vi "TracePartialSnap.vi"() -> ()   [LabVIEW 2012]
uses:
  <vilib>/userdefined/High Color/IMAQdx.ctl
  <vilib>/vision/driver/NI_Vision_Acquisition_Software.lvlib
  <vilib>/vision/NI_Vision_Development_Module.lvlib
panel:
  out "Array":i32[](array[numeric])
  out "Image Out":T1(plugin-control)
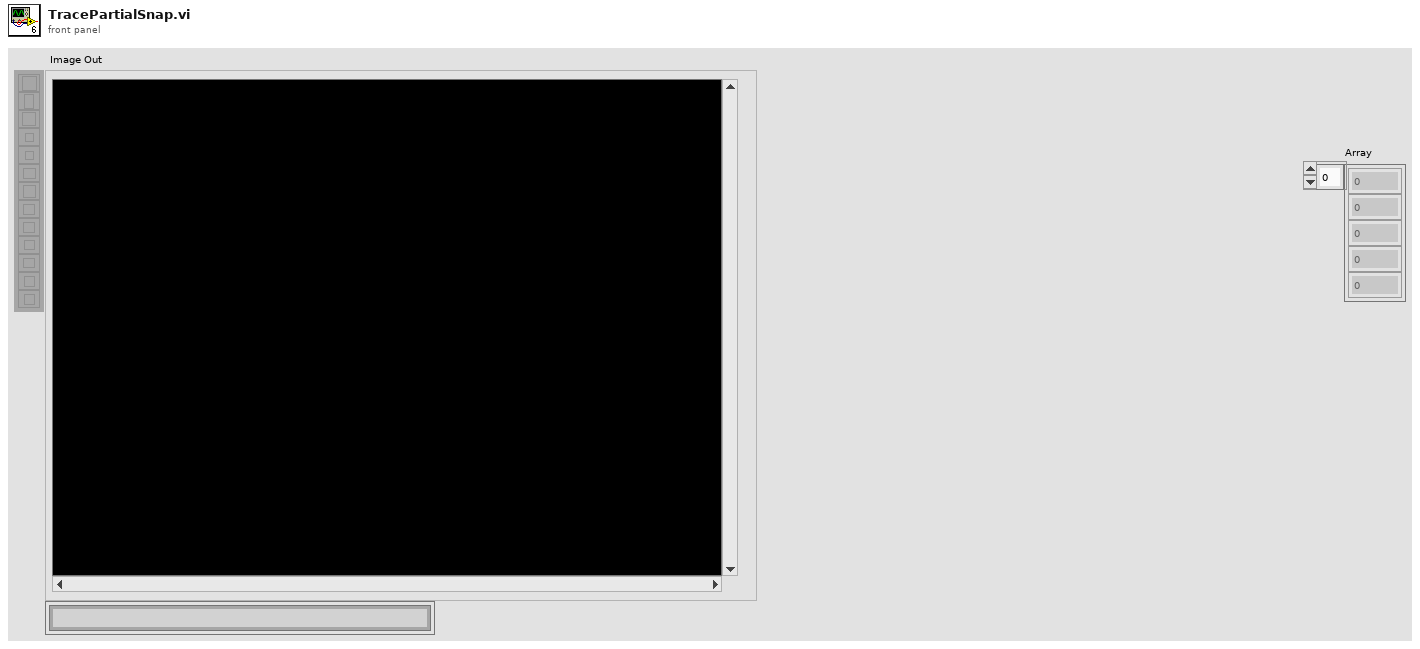
[diagram p1: front panel]
types:
  T1 = typedef "IMAQ Image.ctl" = refnum<image>
  T2 = typedef "Image Type" = u32
  T3 = typedef "IMAQdx.ctl" = refnum<k21>
  T4 = cluster{"Position":cluster{"x":sgl, "y":sgl}, "Angle":sgl, "Scale":sgl, "Score":sgl, "Bounding Box":cluster{"x":sgl, "y":sgl}[]}[]
  T5 = cluster{"Matches (Pattern Matching 1)[0]":cluster{"Position":cluster{"x":sgl, "y":sgl}, "Angle":sgl, "Scale":sgl, "Score":sgl, "Bounding Box":cluster{"x":sgl, "y":sgl}[]}, "Matches (Pattern Matching 1)[1]":cluster{"Position":cluster{"x":sgl, "y":sgl}, "Angle":sgl, "Scale":sgl, "Score":sgl, "Bounding Box":cluster{"x":sgl, "y":sgl}[]}, "Matches (Pattern Matching 1)[2]":cluster{"Position":cluster{"x":sgl, "y":sgl}, "Angle":sgl, "Scale":sgl, "Score":sgl, "Bounding Box":cluster{"x":sgl, "y":sgl}[]}, "Matches (Pattern Matching 1)[3]":cluster{"Position":cluster{"x":sgl, "y":sgl}, "Angle":sgl, "Scale":sgl, "Score":sgl, "Bounding Box":cluster{"x":sgl, "y":sgl}[]}}
  T6 = cluster{"Bounding Box[0]":cluster{"x":sgl, "y":sgl}, "Bounding Box[1]":cluster{"x":sgl, "y":sgl}, "Bounding Box[2]":cluster{"x":sgl, "y":sgl}, "Bounding Box[3]":cluster{"x":sgl, "y":sgl}, "Bounding Box[4]":cluster{"x":sgl, "y":sgl}, "Bounding Box[5]":cluster{"x":sgl, "y":sgl}, "Bounding Box[6]":cluster{"x":sgl, "y":sgl}, "Bounding Box[7]":cluster{"x":sgl, "y":sgl}, "Bounding Box[8]":cluster{"x":sgl, "y":sgl}}
  T7 = cluster{"[0]":i32, "[1]":i32, "[2]":i32, "[3]":i32}
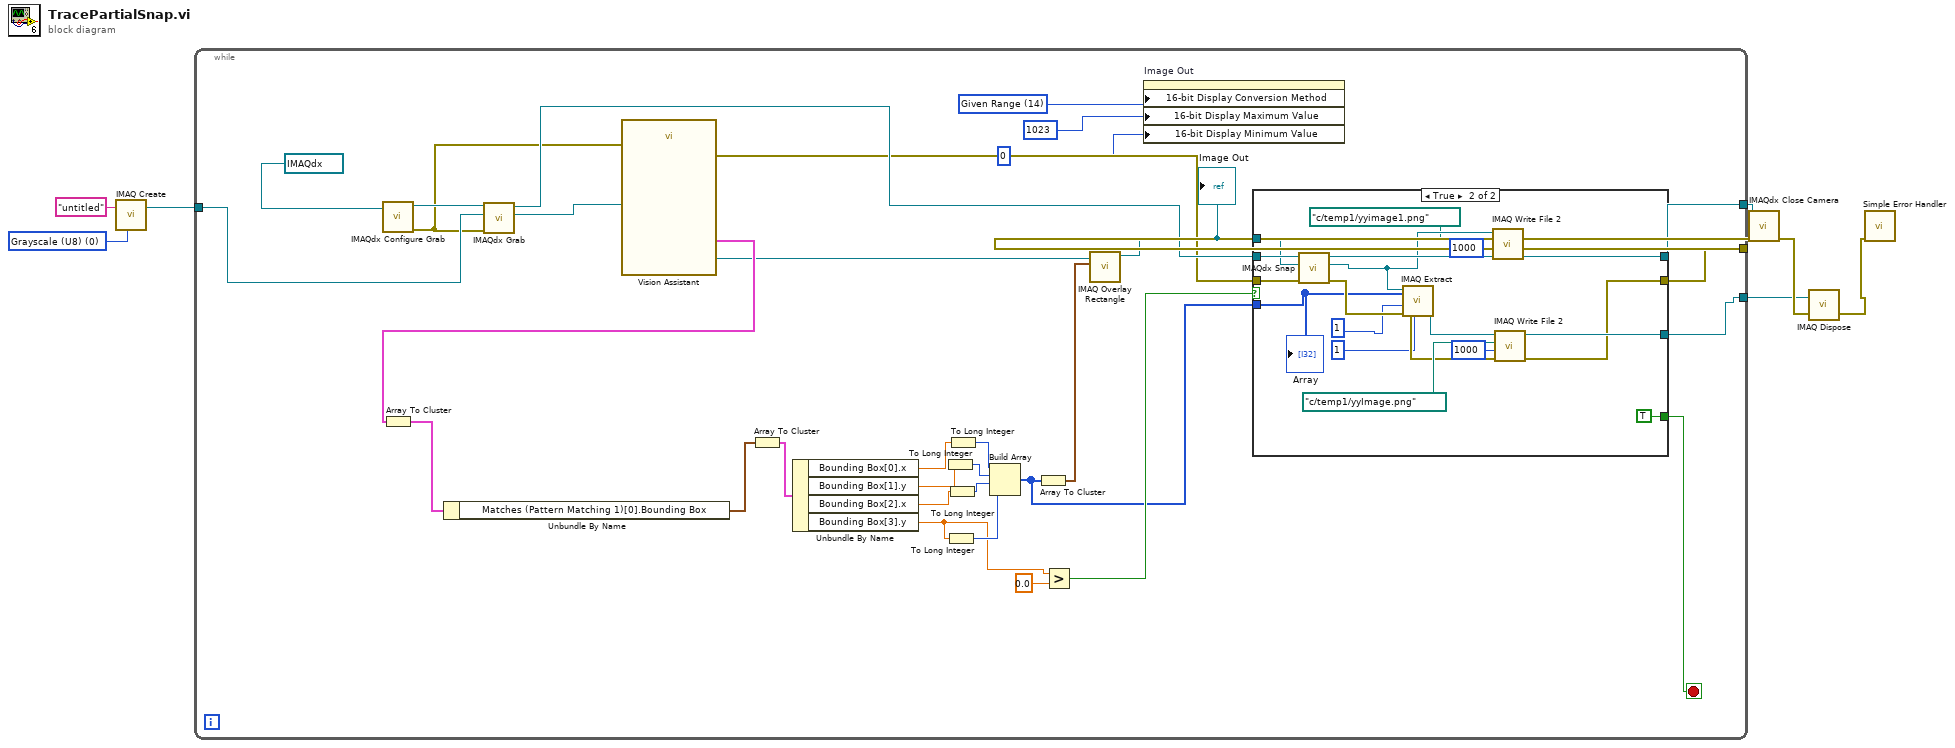
[diagram p0: block diagram]
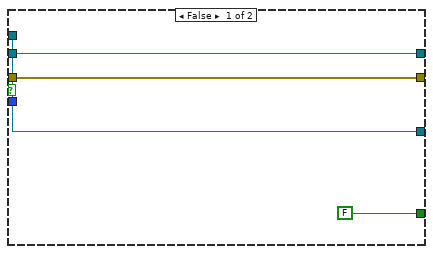
[diagram p2: hidden frame]
diagram:
  w7 = T2 0 items=["Grayscale (U8)", "Grayscale (I16)", "Grayscale (SGL)", "Complex (CSG)", "RGB (U32)", "HSL (U32)", "RGB (U64)", "Grayscale (U16)"] ("Image Type")
  n1 = call "IMAQ Create"("Image Name"="untitled", "Image Type"=w7) -> ("New Image"=w6:T1)  [unwired: 3 in, 1 out]
  n2 = while {
    tunnel: w6 -> [w39]
    tunnel: [w27] -> w3
    tunnel: [w25] -> w2
    tunnel: [w23] -> w1
    stop <- w22 stop-if-true
    w20 = u32 14 items=["Default"=10, "Most Significant Bits"=11, "Full Dynamic"=12, "Downshift"=13, "Given Range"=14, "90% Dynamic"=15, "Given Percent Range"=16] ("16-bit Display Mapping:Conversion Method")
    n3 = call <vilib>:"IMAQdx Configure Grab.vi"("Session In"=T3 "cam0") -> ("error out"=w21:errorcluster, "Session Out"=w40:T3)  [unwired: 9 in]
    n4 = call <vilib>:"IMAQdx Grab.vi"("error in"=w21, "Image In"=w39, "Session In"=w40) -> ("Image Out"=w38:T1, "Session Out"=w28:T3)  [unwired: 5 in, 2 out]
    n5 = call "Vision Assistant"("Image In"=w38, "error in"=w21) -> ("Image Out"=w32:T1, "Matches (Pattern Matching 1)"=w33:T4, "error out"=w26:errorcluster)  [unwired: 23 in]
    n6 = Array To Cluster(array=w33) -> (cluster=w37:T5)
    n7 = Unbundle By Name(w37) -> ("Matches (Pattern Matching 1)[0].Bounding Box"=w36:cluster{"x":sgl, "y":sgl}[])
    n8 = Array To Cluster(array=w36) -> (cluster=w35:T6)
    n9 = Unbundle By Name(w35) -> ("Bounding Box[0].x"=w16:sgl, "Bounding Box[1].y"=w13:sgl, "Bounding Box[2].x"=w10:sgl, "Bounding Box[3].y"=w9:sgl)
    n10 = To Long Integer(number=w13) -> (32bit integer=w14:i32)
    n11 = To Long Integer(number=w9) -> (32bit integer=w12:i32)
    n12 = To Long Integer(number=w10) -> (32bit integer=w11:i32)
    n13 = To Long Integer(number=w16) -> (32bit integer=w15:i32)
    n14 = Build Array(w15, w14, w11, w12) -> (w17:i32[])
    n15 = Array To Cluster(array=w17) -> (cluster=w34:T7)
    n16 = Greater?(x=w9, y=sgl 0.0) -> (0:w29:bool)
    n17 = call "IMAQ Overlay Rectangle"("Rectangle"=w34, "Image"=w32) -> ("Image Out"=w24:T1)  [unwired: 8 in, 1 out]
    "Image Out" <- w24
    n18 = property on="Image Out" class="ImageControl"("16-bit Display Conversion Method"=w20, "16-bit Display Maximum Value"=1023 ("16-bit Display Mapping:Maximum Value"), "16-bit Display Minimum Value"=0 ("16-bit Display Mapping:Minimum Value")) -> ()  [unwired: 2 in, 2 out]
    n19 = case shown="True" w29 {
      tunnel: w28 -> [w44 w62]
      tunnel: [w44 w61] -> w27
      tunnel: w26 -> [w43 w60]
      tunnel: [w43 w55] -> w25
      tunnel: w24 -> [w42 w59]
      tunnel: [w42 w56] -> w23
      tunnel: [FALSE TRUE] -> w22
      tunnel: w17 -> [_ w48]
      frame False {
      }
      frame True {
        n20 = call <vilib>:"IMAQdx Snap.vi"("error in"=w60, "Image In"=w59, "Session In"=w62) -> ("error out"=w52:errorcluster, "Image Out"=w47:T1, "Session Out"=w61:T3)  [unwired: 6 in]
        n21 = call "IMAQ Extract"("Y Step Size"=1, "Optional Rectangle"=w48, "error in (no error)"=w52, "X Step Size"=1, "Image Src"=w47) -> ("error out"=w51:errorcluster, "Image Dst Out"=w53:T1)  [unwired: 5 in]
        n22 = call-poly "IMAQ Write File 2"("Image Quality"=u32 1000, "File Path"=path "c:/temp1/yyimage1.png", "Image"=w47) -> ()  [unwired: 7 in, 2 out]
        n23 = call-poly "IMAQ Write File 2"("error in (no error)"=w51, "Image Quality"=u32 1000, "File Path"=path "c:/temp1/yyImage.png", "Image"=w53) -> ("error out"=w55:errorcluster, "Image Out (duplicate)"=w56:T1)  [unwired: 6 in]
        "Array" <- w48
      }
    }
  }
  n24 = call <vilib>:"IMAQdx Close Camera.vi"("error in"=w2, "Session In"=w3) -> ("error out"=w5:errorcluster)  [unwired: 9 in]
  n25 = call "IMAQ Dispose"("Image"=w1, "error in (no error)"=w5) -> ("error out"=w4:errorcluster)  [unwired: 1 in, 3 out]
  n26 = call <vilib>:"Simple Error Handler.vi"("error in (no error)"=w4) -> ()  [unwired: 1 in, 8 out]
